vi "Hand Sign Recognition.vi"() -> ()   [LabVIEW 2022 SP3]
uses:
  System.Speech
  <vilib>/vision/NI_Vision_Development_Module.lvlib
panel:
  out "?":bool
  out "?":bool
  out "?":bool
  out "?":bool
  in  "File Path 2":path
  out "Read String":string
  out "Image":T1(plugin-control)
  in  "File Path":path
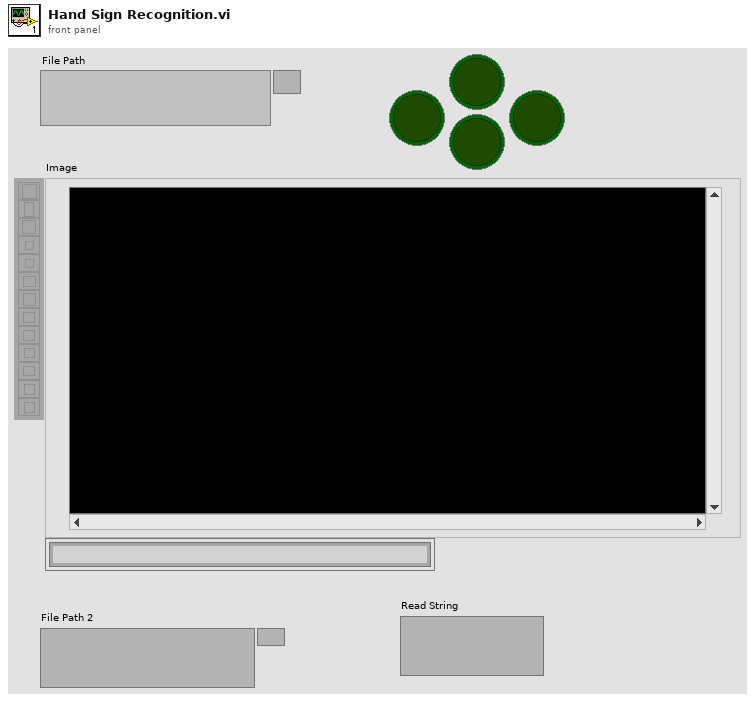
[diagram p1: front panel]
types:
  T1 = typedef "IMAQ Image.ctl" = refnum<image>
  T2 = typedef "Image Type" = u32
  T3 = typedef "IMAQ OCR Session.ctl" = refnum<k1>
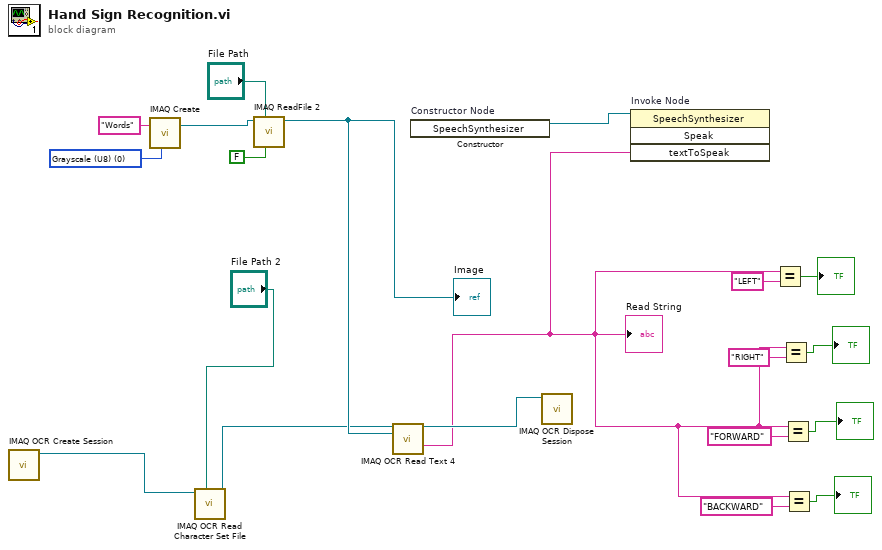
[diagram p0: block diagram]
diagram:
  w19 = T2 0 items=["Grayscale (U8)", "Grayscale (I16)", "Grayscale (SGL)", "Complex (CSG)", "RGB (U32)", "HSL (U32)", "RGB (U64)", "Grayscale (U16)"] ("Image Type")
  n1 = call "IMAQ OCR Create Session"() -> ("IMAQ OCR Session"=w15:T3)  [unwired: 10 in, 1 out]
  n2 = call "IMAQ Create"("Image Name"="Words", "Image Type"=w19) -> ("New Image"=w18:T1)  [unwired: 3 in, 1 out]
  n3 = call "IMAQ OCR Read Character Set File"("File Path"="File Path 2", "IMAQ OCR Session"=w15) -> ("IMAQ OCR Session (dup)"=w13:T3)  [unwired: 7 in, 2 out]
  n4 = call "IMAQ ReadFile 2"("Use File Path Image Type"=FALSE, "File Path"="File Path", "Image"=w18) -> ("Image Out"=w14:T1)  [unwired: 4 in, 4 out]
  "Image" <- w14
  n5 = call "IMAQ OCR Read Text 4"("IMAQ OCR Session"=w13, "Image"=w14) -> ("IMAQ OCR Session (dup)"=w12:T3, "Read String"=w5:string)  [unwired: 7 in, 5 out]
  "Read String" <- w5
  n6 = constructor on="Constructor Node" class="SpeechSynthesizer"() -> (reference out=w10:refnum<k24>)  [unwired: 3 in, 2 out]
  n7 = call "IMAQ OCR Dispose Session"("IMAQ OCR Session"=w12) -> ()  [unwired: 10 in, 1 out]
  n8 = invoke on="Invoke Node" class="SpeechSynthesizer" method="Speak"(reference=w10, "textToSpeak"=w5) -> ()  [unwired: 2 in, 4 out]
  n9 = Equal?(x=w5, y="LEFT") -> (x = y?=→"?":bool)
  n10 = Equal?(x=w5, y="RIGHT") -> (x = y?=→"?":bool)
  n11 = Equal?(x=w5, y="FORWARD") -> (x = y?=→"?":bool)
  n12 = Equal?(x=w5, y="BACKWARD") -> (x = y?=→"?":bool)
